vi "Man_Init.vi"(8 "error in (no error)":errorcluster caption="错误输入（无错误）", 11 "ManUIref":T2) -> (0 "error out":errorcluster caption="错误输出", 3 "DevState":T1={"Type"=41, "Index"=0, "DeviceOpen"=FALSE, "Ch0Start"=FALSE, "Ch1Start"=FALSE} {"Index" items=["0", "1", "2", "3", "4", "5", "6", "7", "8"]; "Type" items=["USBCANFD-200U"=41, "USBCANFD-100U"=42]})   [LabVIEW 2018, in "CAN FD.lvlib"]
uses:
  CAN FD.lvlib
  Typedef/ManUIref.ctl
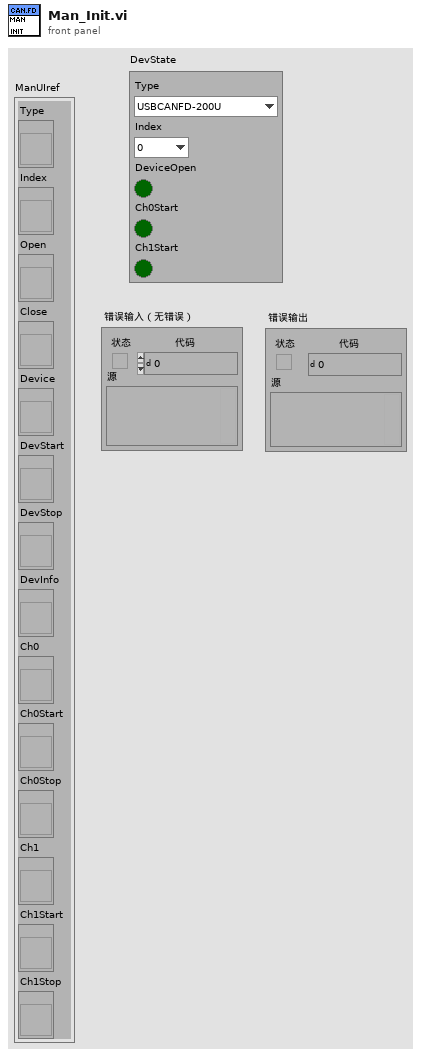
[diagram p1: front panel]
types:
  T1 = cluster{"Type":u32, "Index":u32, "DeviceOpen":bool, "Ch0Start":bool, "Ch1Start":bool}
  T2 = typedef "CAN FD.lvlib/ManUIref.ctl" = cluster{"Type":refnum<vi>, "Index":refnum<vi>, "Open":refnum<vi>, "Close":refnum<vi>, "Device":refnum<vi>, "DevStart":refnum<vi>, "DevStop":refnum<vi>, "DevInfo":refnum<vi>, "Ch0":refnum<vi>, "Ch0Start":refnum<vi>, "Ch0Stop":refnum<vi>, "Ch1":refnum<vi>, "Ch1Start":refnum<vi>, "Ch1Stop":refnum<vi>}
  T3 = typedef "CAN FD.lvlib/CurrentDev.ctl" = cluster{"Type":u32, "Index":u32}
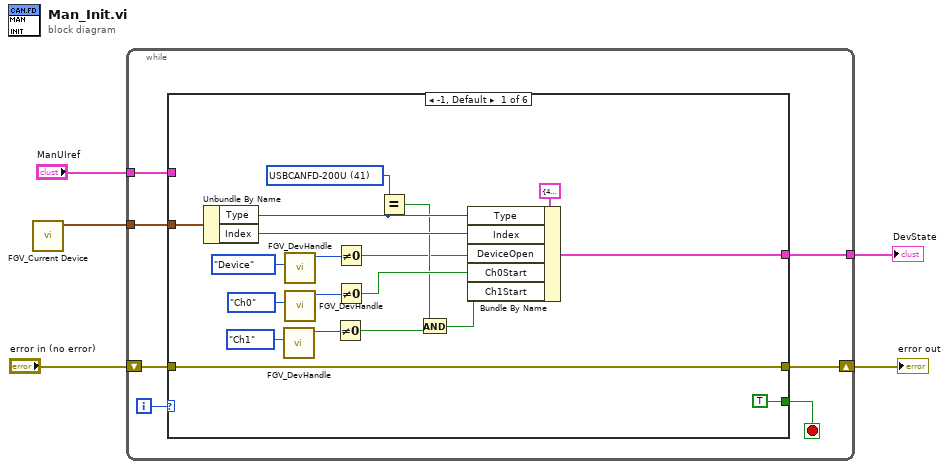
[diagram p0: block diagram]
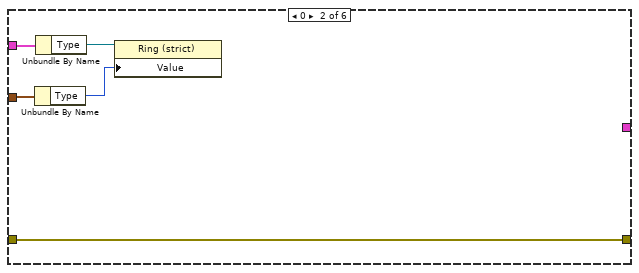
[diagram p2: hidden frame]
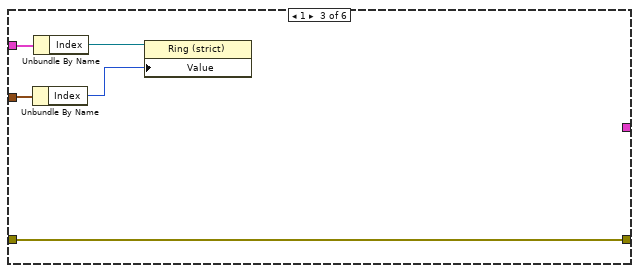
[diagram p3: hidden frame]
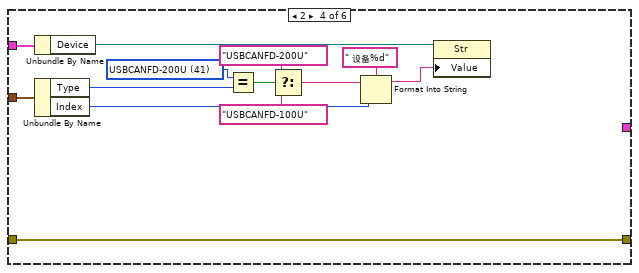
[diagram p4: hidden frame]
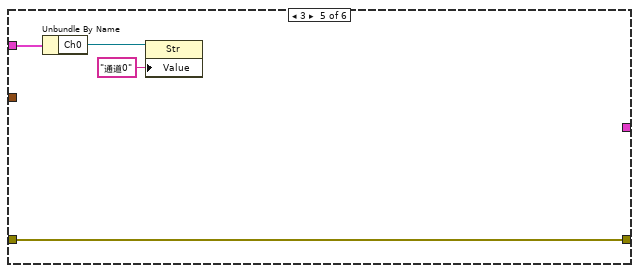
[diagram p5: hidden frame]
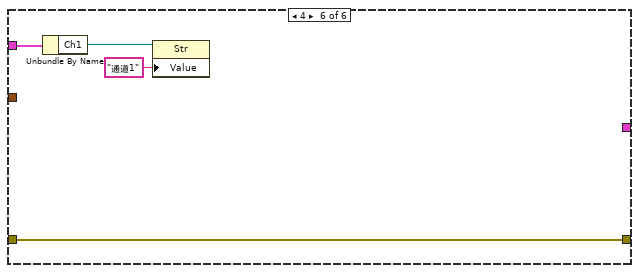
[diagram p6: hidden frame]
diagram:
  n1 = call "FGV_Current Device.vi"() -> ("CurrentDev out"=w2:T3)  [unwired: 10 in, 1 out]
  n2 = while {
    shift-right: [w10] -> w5
    shift-left: "error in (no error)" -> [w9]
    tunnel: "ManUIref" -> [w8]
    tunnel: w2 -> [w7]
    tunnel: [w6] -> w1
    i -> [w12]
    stop <- w11 stop-if-true
    n3 = case shown="-1, Default" w12 {
      tunnel: [TRUE _ _ _ _ _] -> w11
      tunnel: [w30 w36 w41 w54 w58 w62] -> w10
      tunnel: w9 -> [w30 w36 w41 w54 w58 w62]
      tunnel: w8 -> [_ w35 w40 w53 w57 w61]
      tunnel: w7 -> [w29 w33 w38 w51 _ _]
      tunnel: [w16 _ _ _ _ _] -> w6
      frame -1, Default {
        w20 = u32 41 items=["USBCANFD-200U"=41, "USBCANFD-100U"=42] ("Type")
        n4 = Unbundle By Name(w29) -> ("Type"=w21:u32, "Index"=w27:u32)
        n5 = call "FGV_DevHandle.vi"("Type"=enum16{"Device", "Ch0", "Ch1"}."Ch1") -> ("handle out"=w24:u64)  [unwired: 8 in, 2 out]
        n6 = call "FGV_DevHandle.vi"("Type"=enum16{"Device", "Ch0", "Ch1"}."Device") -> ("handle out"=w14:u64)  [unwired: 8 in, 2 out]
        n7 = call "FGV_DevHandle.vi"("Type"=enum16{"Device", "Ch0", "Ch1"}."Ch0") -> ("handle out"=w26:u64)  [unwired: 8 in, 2 out]
        n8 = Not Equal To 0?(x=w24) -> (x != 0?=w18:bool)
        n9 = Not Equal To 0?(x=w14) -> (x != 0?=w13:bool)
        n10 = Not Equal To 0?(x=w26) -> (x != 0?=w25:bool)
        n11 = Equal?(x=w20, y=w21) -> (x = y?=w19:bool)
        n12 = And(x=w19, y=w18) -> (x .and. y?=w17:bool)
        n13 = Bundle By Name(cluster=T1 {"Type"=41, "Index"=0, "DeviceOpen"=FALSE, "Ch0Start"=FALSE, "Ch1Start"=FALSE} ("DevState"), "Type"=w21, "Index"=w27, "DeviceOpen"=w13, "Ch0Start"=w25, "Ch1Start"=w17) -> (w16:T1)
      }
      frame 0 {
        n14 = Unbundle By Name(w33) -> ("Type"=w32:u32)
        n15 = Unbundle By Name(w35) -> ("Type"=w34:refnum<vi>)
        n16 = property class="Ring (strict)"(reference=w34, "Value"=w32) -> ()  [unwired: 1 in, 2 out]
      }
      frame 1 {
        n17 = Unbundle By Name(w38) -> ("Index"=w37:u32)
        n18 = Unbundle By Name(w40) -> ("Index"=w39:refnum<vi>)
        n19 = property class="Ring (strict)"(reference=w39, "Value"=w37) -> ()  [unwired: 1 in, 2 out]
      }
      frame 2 {
        w49 = u32 41 items=["USBCANFD-200U"=41, "USBCANFD-100U"=42] ("Type")
        n20 = Unbundle By Name(w53) -> ("Device"=w52:refnum<vi>)
        n21 = Unbundle By Name(w51) -> ("Type"=w50:u32, "Index"=w44:u32)
        n22 = Equal?(x=w49, y=w50) -> (x = y?=w48:bool)
        n23 = Select(t="USBCANFD-200U", s=w48, f="USBCANFD-100U") -> (s? t:f=w45:string)
        n24 = Format Into String(format string=" 设备%d" ("格式字符串"), initial string=w45, w44) -> (resulting string=w42:string)  [unwired: 1 in, 1 out]
        n25 = property class="Str"(reference=w52, "Value"=w42) -> ()  [unwired: 1 in, 2 out]
      }
      frame 3 {
        n26 = Unbundle By Name(w57) -> ("Ch0"=w56:refnum<vi>)
        n27 = property class="Str"(reference=w56, "Value"="通道0" ("值")) -> ()  [unwired: 1 in, 2 out]
      }
      frame 4 {
        n28 = Unbundle By Name(w61) -> ("Ch1"=w60:refnum<vi>)
        n29 = property class="Str"(reference=w60, "Value"="通道1" ("值")) -> ()  [unwired: 1 in, 2 out]
      }
    }
  }
  "error out" <- w5
  "DevState" <- w1
